vi "DataGraph_MouseMove.vi"(7 "Boundary":T1, 8 "error in (no error)":errorcluster, 9 "Coords":T2, 10 "Raw Coords":T2, 11 "Mass_Graph":refnum<vi>) -> (0 "error out":errorcluster)   [LabVIEW 2018, in "DataGraphXControl.xctl"]
uses:
  DataGraphXControl.xctl
  <vilib>/Utility/miscctls.llb/LVPoint32TypeDef.ctl
panel:
  out "Value":cluster{"X":dbl[], "Y":dbl[]}
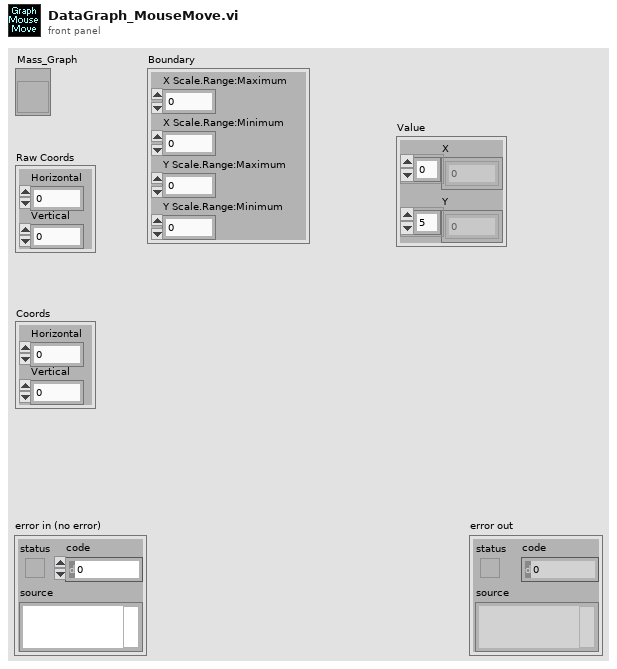
[diagram p1: front panel]
types:
  T1 = cluster{"X Scale.Range:Maximum":dbl, "X Scale.Range:Minimum":dbl, "Y Scale.Range:Maximum":dbl, "Y Scale.Range:Minimum":dbl}
  T2 = typedef "LVPoint32TypeDef.ctl" = cluster{"Horizontal":i32, "Vertical":i32}
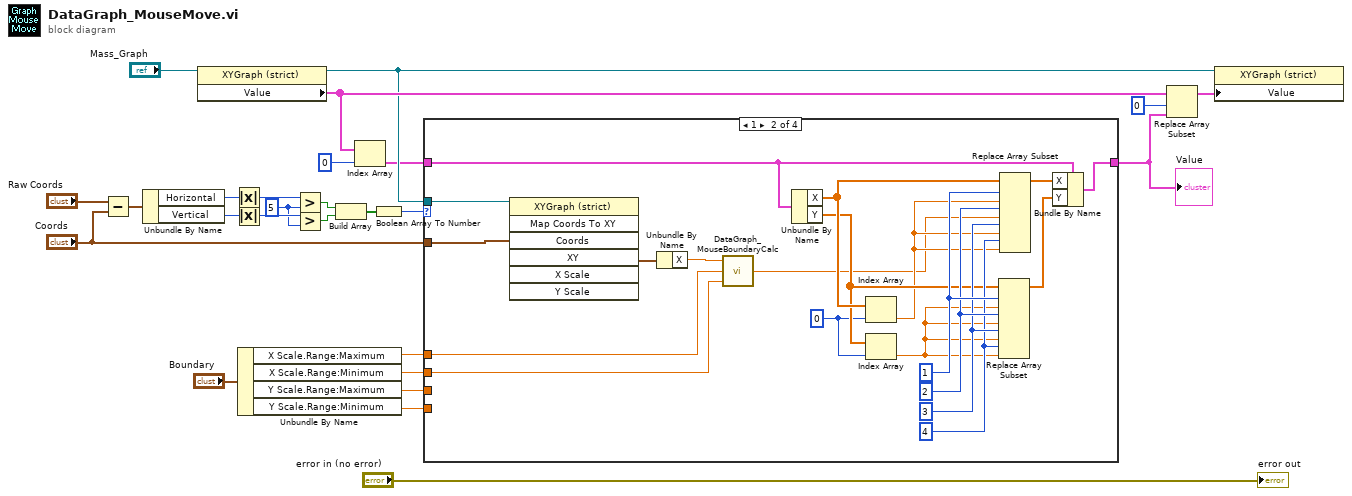
[diagram p0: block diagram]
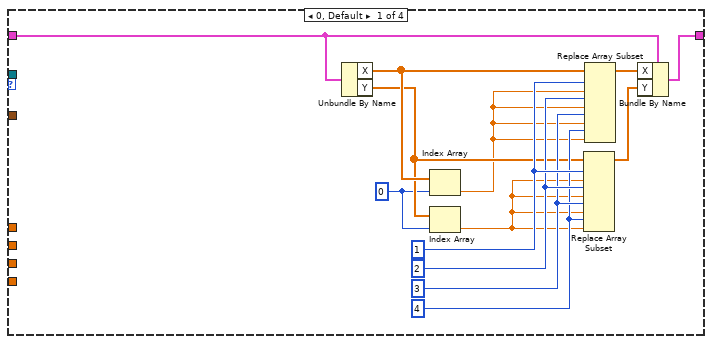
[diagram p2: hidden frame]
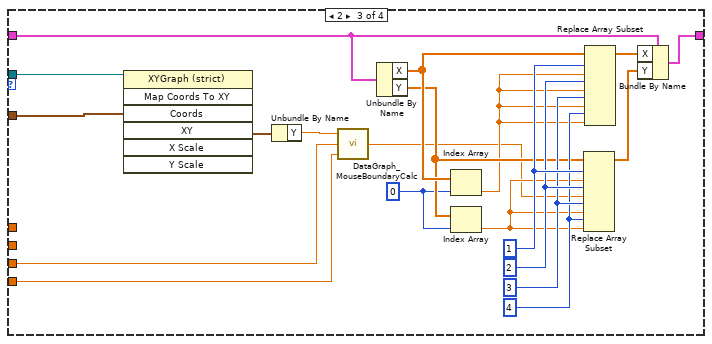
[diagram p3: hidden frame]
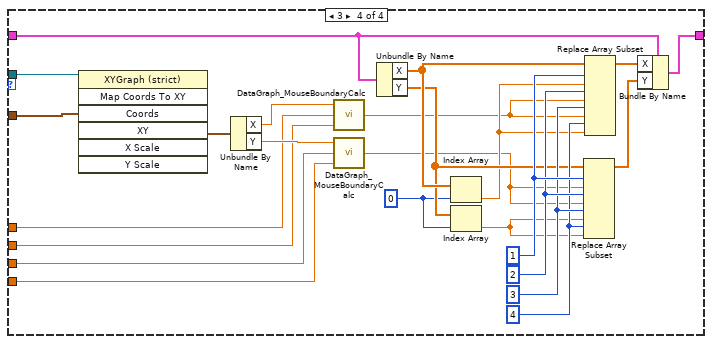
[diagram p4: hidden frame]
diagram:
  w17 = 5 ("y")
  n1 = Subtract(x="Raw Coords", y="Coords") -> (x-y=w22:T2)
  n2 = Unbundle By Name(w22) -> ("Horizontal"=w21:i32, "Vertical"=w20:i32)
  n3 = property class="XYGraph (strict)"(reference="Mass_Graph") -> (reference out=w8:refnum<vi>, "Value"=w9:cluster{"X":dbl[], "Y":dbl[]}[])  [unwired: 1 in, 1 out]
  n4 = Absolute Value(x=w21) -> (abs(x)=w19:i32)
  n5 = Absolute Value(x=w20) -> (abs(x)=w18:i32)
  n6 = Unbundle By Name("Boundary") -> ("X Scale.Range:Maximum"=w4:dbl, "X Scale.Range:Minimum"=w3:dbl, "Y Scale.Range:Maximum"=w2:dbl, "Y Scale.Range:Minimum"=w1:dbl)
  n7 = Greater?(x=w19, y=w17) -> (0:w15:bool)
  n8 = Greater?(x=w18, y=w17) -> (0:w14:bool)
  n9 = Build Array(w15, w14) -> (w13:bool[])
  n10 = Index Array(array=w9, index=0) -> (element=w7:cluster{"X":dbl[], "Y":dbl[]})
  n11 = Boolean Array To Number(Boolean array=w13) -> (number=w12:u32)
  n12 = case shown="1" w12 {
    tunnel: "Coords" -> [_ w59 w79 w103]
    tunnel: w8 -> [_ w58 w78 w102]
    tunnel: w7 -> [w30 w47 w67 w89]
    tunnel: [w29 w46 w66 w88] -> w6
    tunnel: w4 -> [_ w41 _ w83]
    tunnel: w3 -> [_ w40 _ w82]
    tunnel: w2 -> [_ _ w61 w81]
    tunnel: w1 -> [_ _ w60 w80]
    frame 0, Default {
      w33 = 0 ("index")
      w36 = 4 ("index")
      w37 = 3 ("index")
      w38 = 2 ("index")
      w39 = 1 ("index")
      n13 = Unbundle By Name(w30) -> ("X"=w35:dbl[], "Y"=w34:dbl[])
      n14 = Index Array(array=w35, index=w33) -> (element=w28:dbl)
      n15 = Index Array(array=w34, index=w33) -> (element=w27:dbl)
      n16 = Replace Array Subset(array=w34, new element #1=w27, index #1=w39, new element #2=w27, index #2=w38, new element #3=w27, index #3=w37, new element #4=w27, index #4=w36) -> (w31:dbl[])
      n17 = Replace Array Subset(array=w35, new element #1=w28, index #1=w39, new element #2=w28, index #2=w38, new element #3=w28, index #3=w37, new element #4=w28, index #4=w36) -> (w32:dbl[])
      n18 = Bundle By Name(cluster=w30, "X"=w32, "Y"=w31) -> (w29:cluster{"X":dbl[], "Y":dbl[]})
    }
    frame 1 {
      w50 = 0 ("index")
      w53 = 4 ("index")
      w54 = 3 ("index")
      w55 = 2 ("index")
      w56 = 1 ("index")
      n19 = invoke class="XYGraph (strict)" method="Map Coords To XY"(reference=w58, "Coords"=w59) -> ("XY"=w57:cluster{"X":dbl, "Y":dbl})  [unwired: 5 in, 6 out]
      n20 = Unbundle By Name(w57) -> ("X"=w43:dbl)
      n21 = call "DataGraph_MouseBoundaryCalc.vi"("Minimum"=w40, "Maximum"=w41, "Value in"=w43) -> ("Value out"=w42:dbl)
      n22 = Unbundle By Name(w47) -> ("X"=w52:dbl[], "Y"=w51:dbl[])
      n23 = Index Array(array=w52, index=w50) -> (element=w45:dbl)
      n24 = Index Array(array=w51, index=w50) -> (element=w44:dbl)
      n25 = Replace Array Subset(array=w51, new element #1=w44, index #1=w56, new element #2=w44, index #2=w55, new element #3=w44, index #3=w54, new element #4=w44, index #4=w53) -> (w48:dbl[])
      n26 = Replace Array Subset(array=w52, new element #1=w45, index #1=w56, new element #2=w42, index #2=w55, new element #3=w45, index #3=w54, new element #4=w45, index #4=w53) -> (w49:dbl[])
      n27 = Bundle By Name(cluster=w47, "X"=w49, "Y"=w48) -> (w46:cluster{"X":dbl[], "Y":dbl[]})
    }
    frame 2 {
      w70 = 0 ("index")
      w73 = 4 ("index")
      w74 = 3 ("index")
      w75 = 2 ("index")
      w76 = 1 ("index")
      n28 = invoke class="XYGraph (strict)" method="Map Coords To XY"(reference=w78, "Coords"=w79) -> ("XY"=w77:cluster{"X":dbl, "Y":dbl})  [unwired: 5 in, 6 out]
      n29 = Unbundle By Name(w77) -> ("Y"=w63:dbl)
      n30 = call "DataGraph_MouseBoundaryCalc.vi"("Minimum"=w60, "Maximum"=w61, "Value in"=w63) -> ("Value out"=w62:dbl)
      n31 = Unbundle By Name(w67) -> ("X"=w72:dbl[], "Y"=w71:dbl[])
      n32 = Index Array(array=w72, index=w70) -> (element=w64:dbl)
      n33 = Index Array(array=w71, index=w70) -> (element=w65:dbl)
      n34 = Replace Array Subset(array=w71, new element #1=w65, index #1=w76, new element #2=w62, index #2=w75, new element #3=w65, index #3=w74, new element #4=w65, index #4=w73) -> (w68:dbl[])
      n35 = Replace Array Subset(array=w72, new element #1=w64, index #1=w76, new element #2=w64, index #2=w75, new element #3=w64, index #3=w74, new element #4=w64, index #4=w73) -> (w69:dbl[])
      n36 = Bundle By Name(cluster=w67, "X"=w69, "Y"=w68) -> (w66:cluster{"X":dbl[], "Y":dbl[]})
    }
    frame 3 {
      w94 = 0 ("index")
      w97 = 4 ("index")
      w98 = 3 ("index")
      w99 = 2 ("index")
      w100 = 1 ("index")
      n37 = invoke class="XYGraph (strict)" method="Map Coords To XY"(reference=w102, "Coords"=w103) -> ("XY"=w101:cluster{"X":dbl, "Y":dbl})  [unwired: 5 in, 6 out]
      n38 = Unbundle By Name(w101) -> ("X"=w87:dbl, "Y"=w85:dbl)
      n39 = call "DataGraph_MouseBoundaryCalc.vi"("Minimum"=w82, "Maximum"=w83, "Value in"=w87) -> ("Value out"=w86:dbl)
      n40 = call "DataGraph_MouseBoundaryCalc.vi"("Minimum"=w80, "Maximum"=w81, "Value in"=w85) -> ("Value out"=w84:dbl)
      n41 = Unbundle By Name(w89) -> ("X"=w96:dbl[], "Y"=w95:dbl[])
      n42 = Index Array(array=w96, index=w94) -> (element=w92:dbl)
      n43 = Index Array(array=w95, index=w94) -> (element=w93:dbl)
      n44 = Replace Array Subset(array=w95, new element #1=w84, index #1=w100, new element #2=w84, index #2=w99, new element #3=w93, index #3=w98, new element #4=w93, index #4=w97) -> (w90:dbl[])
      n45 = Replace Array Subset(array=w96, new element #1=w92, index #1=w100, new element #2=w86, index #2=w99, new element #3=w86, index #3=w98, new element #4=w92, index #4=w97) -> (w91:dbl[])
      n46 = Bundle By Name(cluster=w89, "X"=w91, "Y"=w90) -> (w88:cluster{"X":dbl[], "Y":dbl[]})
    }
  }
  "Value" <- w6
  n47 = Replace Array Subset(array=w9, new element=w6, index=0) -> (w24:cluster{"X":dbl[], "Y":dbl[]}[])
  n48 = property class="XYGraph (strict)"(reference=w8, "Value"=w24) -> ()  [unwired: 1 in, 2 out]
  "error out" <- "error in (no error)"
